vi "test - Clear CSM Queue.vi"(8 "error in (no error)":errorcluster, 11 "TestCase in":refnum<class "testcase-Basic-Function.lvclass">) -> (0 "error out":errorcluster, 3 "TestCase out":refnum<class "testcase-Basic-Function.lvclass">)   [LabVIEW 2017, in "testcase-Basic-Function.lvclass"]
uses:
  testcase-Basic-Function.lvclass
  src/user.lib/_NEVSTOP/Communicable State Machine(CSM)/_Support/CSMQ/_CSMOFGVOPER.ctl
  src/user.lib/_NEVSTOP/Communicable State Machine(CSM)/AdvanceAPI/CSM - Revert Arguments-Safe String.vi
  src/user.lib/_NEVSTOP/Communicable State Machine(CSM)/AdvanceAPI/CSM - Make String Arguments Safe.vi
  src/user.lib/_NEVSTOP/Communicable State Machine(CSM)/AdvanceAPI/CSM - Break Down Multiple States String.vi
  src/user.lib/_NEVSTOP/Communicable State Machine(CSM)/AdvanceAPI/CSM - Compact Multiple States.vi
  src/user.lib/_NEVSTOP/Communicable State Machine(CSM)/AdvanceAPI/CSM - Keywords.vi
  src/user.lib/_NEVSTOP/Communicable State Machine(CSM)/_Shared/Trim Single-line Text.vi
  <vilib>/addons/_JKI Toolkits/VI Tester/TestCase.llb/TestCase.lvclass
  src/user.lib/_NEVSTOP/Communicable State Machine(CSM)/Communicable State Machine.lvlib
  C:/Program Files (x86)/National Instruments/LabVIEW 2017/vi.lib/addons/_JKI Toolkits/VI Tester/TestCase.llb/TestCase.lvclass
panel:
  out "# pending insert":i32
  out "# pending remove":i32
  out "#Flushed":cluster{i32, i32}
  out "#elements in queue":i32
  out "error out 5":errorcluster
  out "error out 4":errorcluster
  out "error out 3":errorcluster
  out "error out 2":errorcluster
  out "error out 1":errorcluster
  out "State History":string
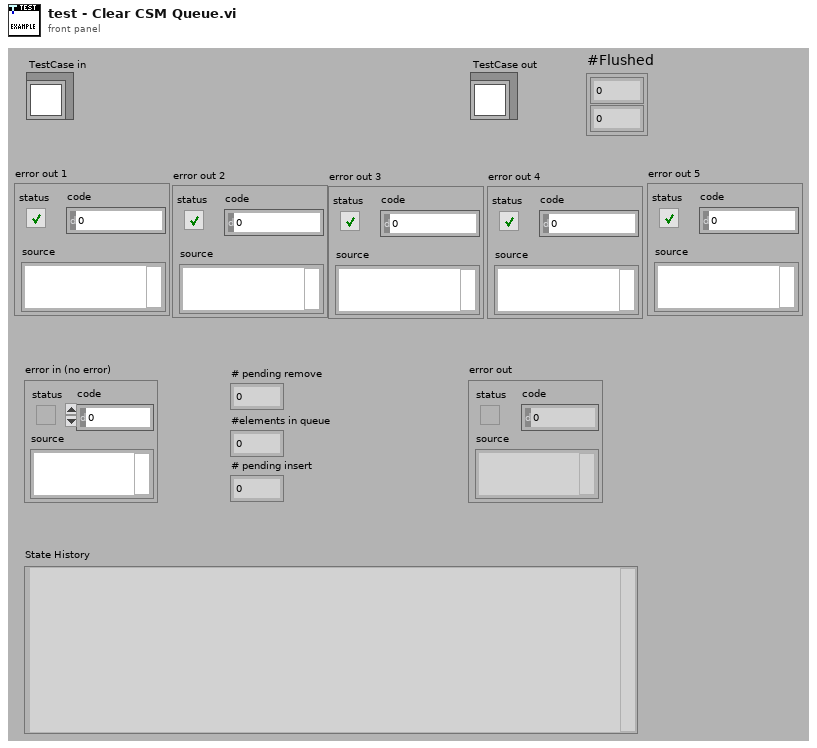
[diagram p1: front panel]
types:
  T1 = enum32{"Invalid", "Standard", "Closed", "Hidden", "Minimized", "Maximized"}
  T2 = enum32{"invalid app kind", "Development System", "Run Time System", "Student Edition", "Embedded LabVIEW", "Evaluation", "Custom"}
  T3 = typedef "Communicable State Machine.lvlib/_CSMOFGVOPER.ctl" = enum16{"Create If not Exist", "Get By Name", "List", "Check If Name Exists", "Release", "Module Status", "Create Status Event Handler", "Destroy Status Event Handler", "Clear Invalid Objs"}
  T4 = typedef "Communicable State Machine.lvlib/_CSM_Response Source Message.ctl" = cluster{"‘State":string, "’Arguments":string, "’Error":errorcluster}
  T5 = cluster{"Current VI Reference":refnum<vi>, "Close Panel on Exit?":bool}
  T6 = cluster{"Core":cluster{"Current VI Reference":refnum<vi>, "Close Panel on Exit?":bool}, "Your Boolean data":bool, "Your string data":string}
  T7 = typedef "Communicable State Machine.lvlib/_CSMObj.ctl" = cluster{"info":T8, "Refs":T10}
  T8 = typedef "Communicable State Machine.lvlib/_CSMObj-Info.ctl" = cluster{"Module Name":string, "Requested Name":string, "Group Name":string, "Mode":T9, "Allowed Messages":string[]}
  T9 = typedef "Communicable State Machine.lvlib/_CSM_MODE.ctl" = enum16{"Not Exist", "Stand Alone", "CSM", "Worker", "Worker Agent", "Chain Node", "Chain"}
  T10 = typedef "Communicable State Machine.lvlib/_CSMObj-Refs.ctl" = cluster{"WatchDogQ":refnum<queue>, "CSMDataDVR":refnum<data-value>, "Queue":T11, "GroupDataDVR":refnum<data-value>, "TagMap":refnum<data-value>, "ExitEvent":refnum<user-event>, "NewStateEvent":refnum<user-event>, "StatusEvent":refnum<user-event>, "InterruptEvent":refnum<user-event>}
  T11 = typedef "Communicable State Machine.lvlib/Priority Queue.ctl" = cluster{"HPriorityQ":refnum<queue>, "LowPriorityQ":refnum<queue>}
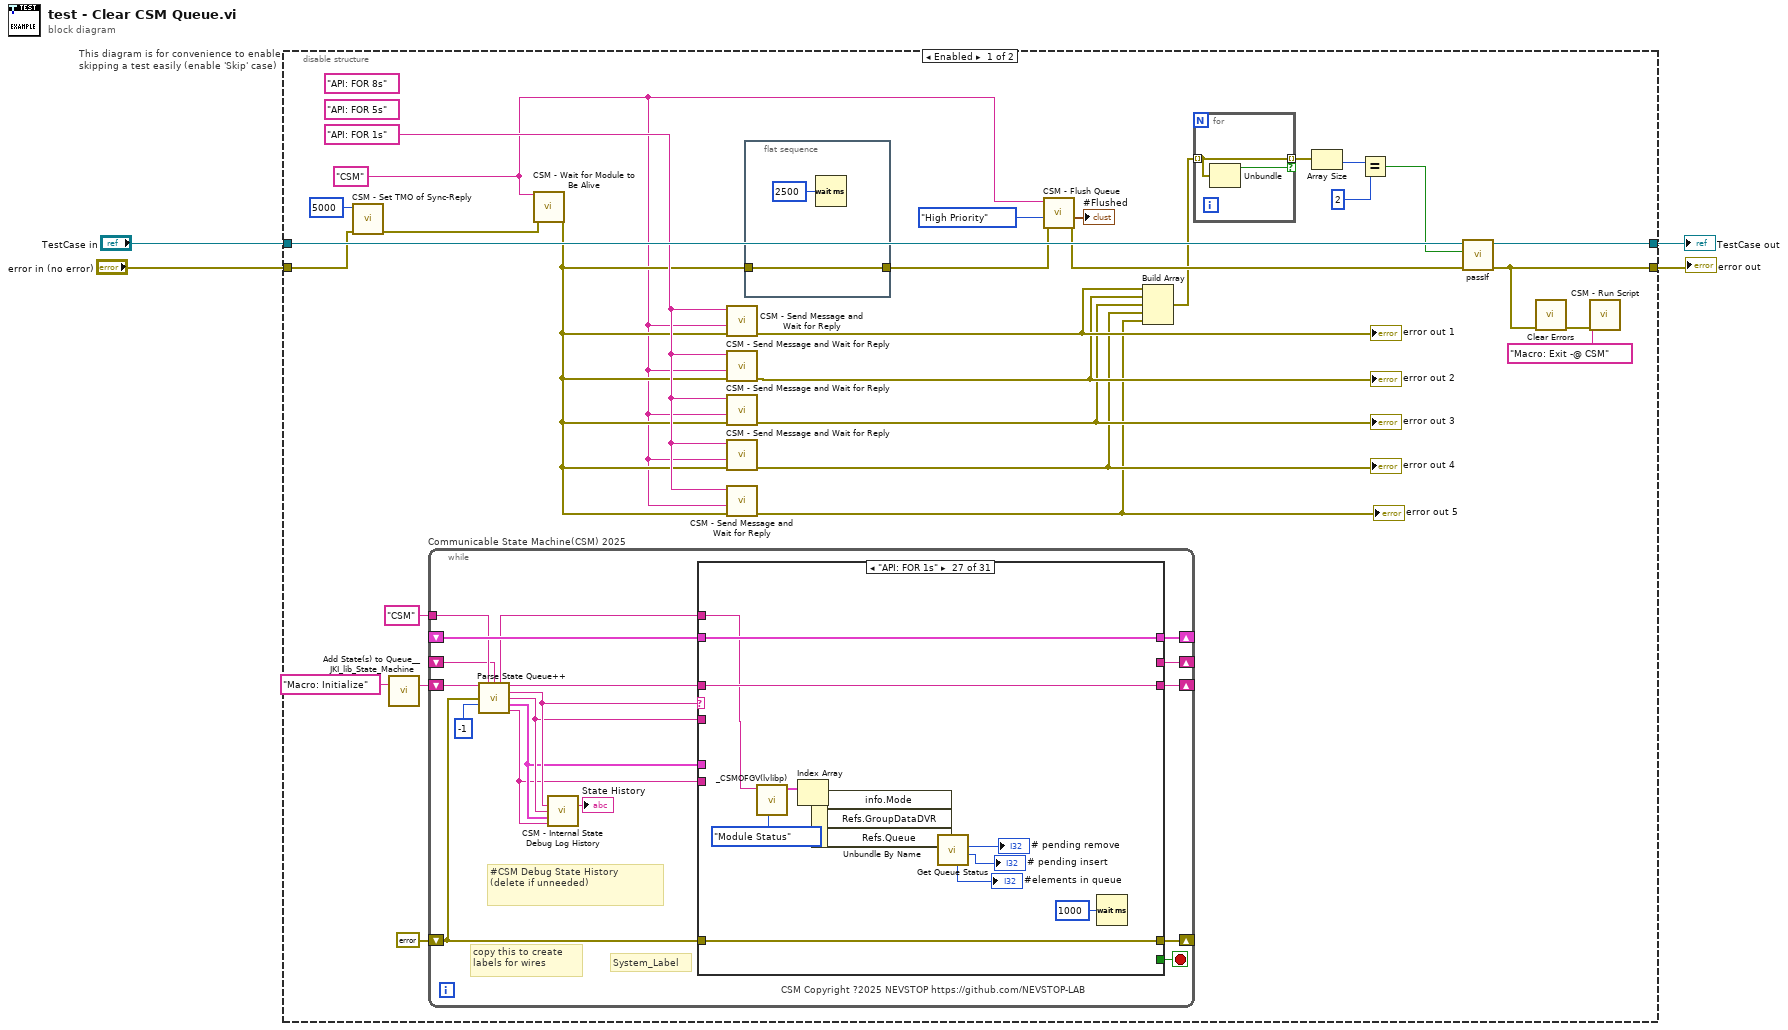
[diagram p0: block diagram]
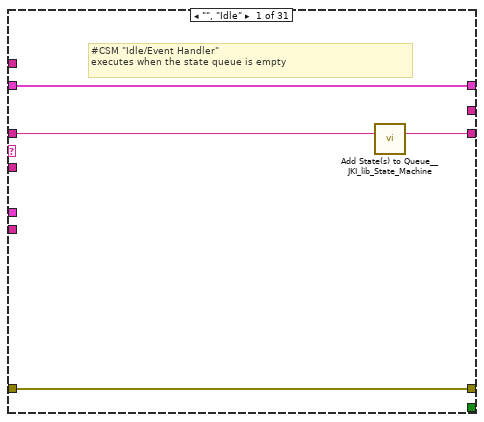
[diagram p2: hidden frame]
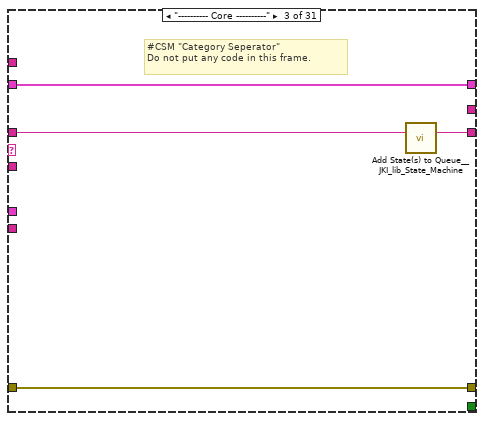
[diagram p4: hidden frame]
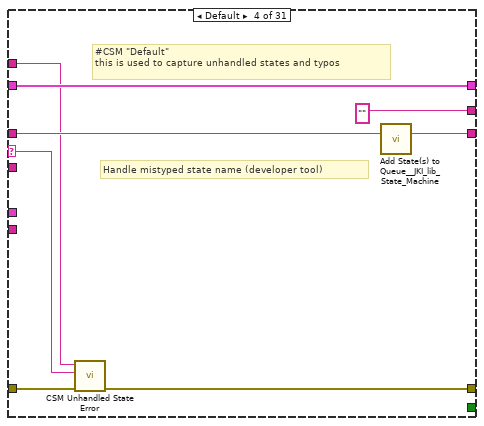
[diagram p5: hidden frame]
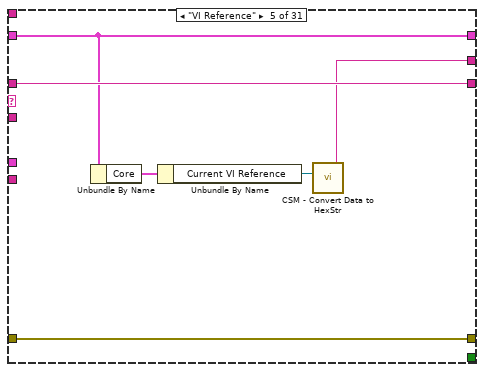
[diagram p6: hidden frame]
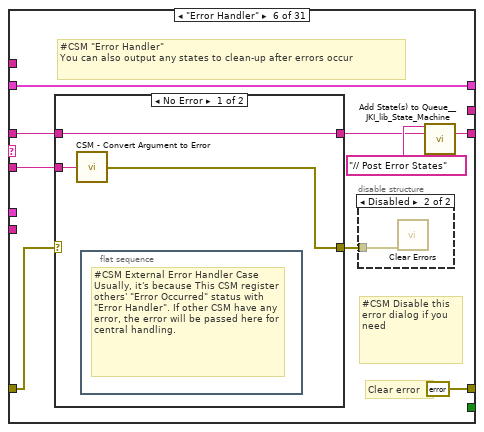
[diagram p7: hidden frame]
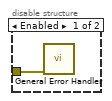
[diagram p8: hidden frame]
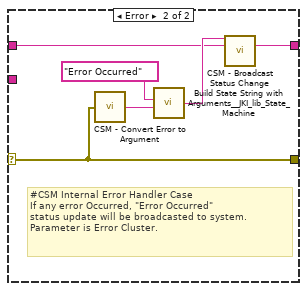
[diagram p9: hidden frame]
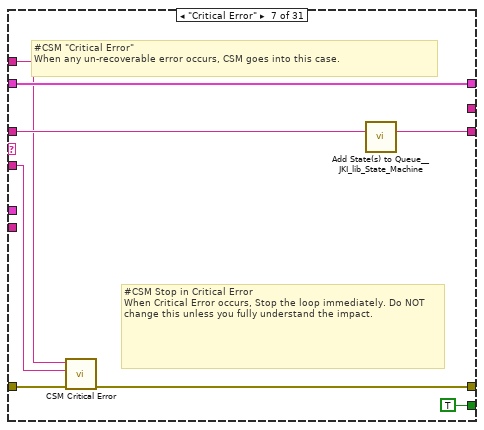
[diagram p10: hidden frame]
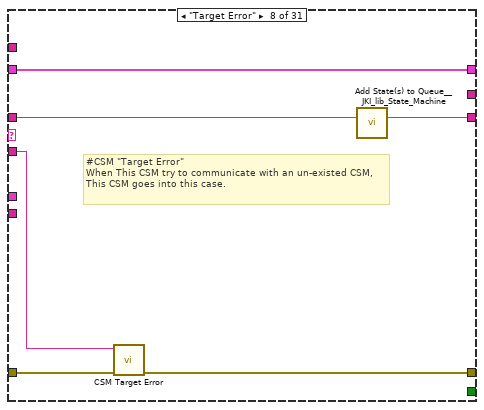
[diagram p11: hidden frame]
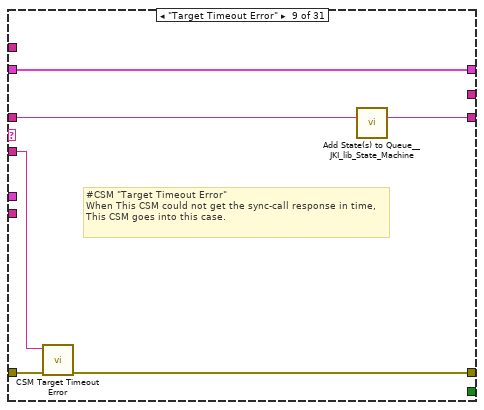
[diagram p12: hidden frame]
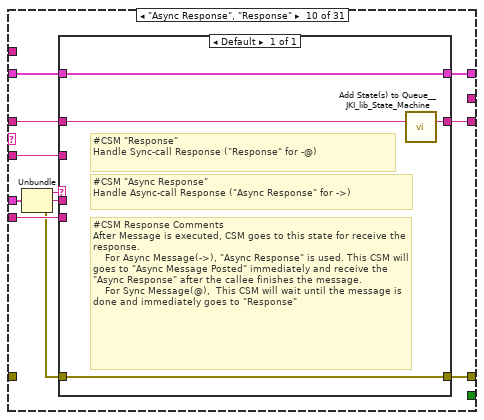
[diagram p13: hidden frame]
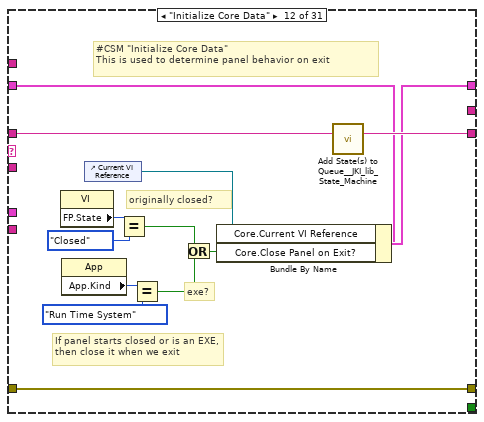
[diagram p15: hidden frame]
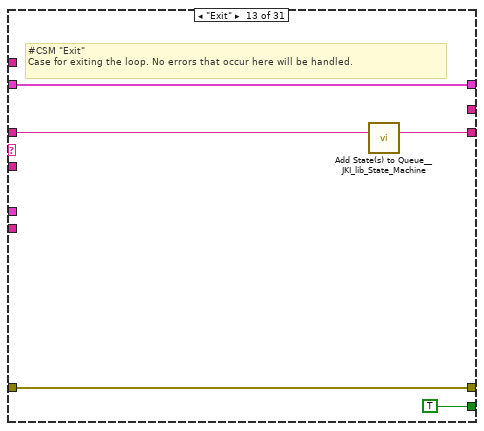
[diagram p16: hidden frame]
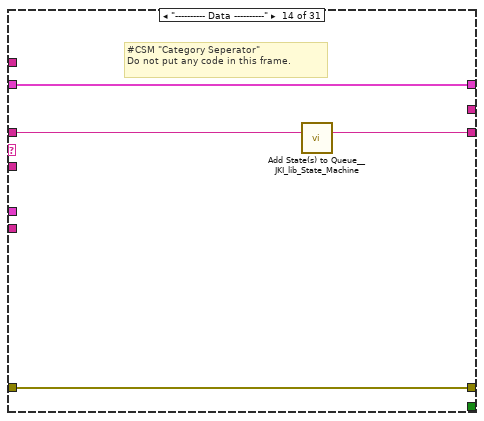
[diagram p17: hidden frame]
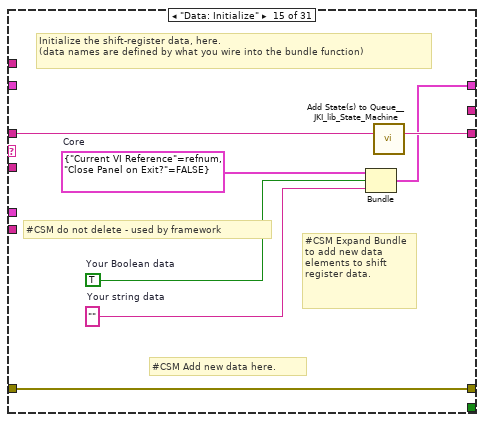
[diagram p18: hidden frame]
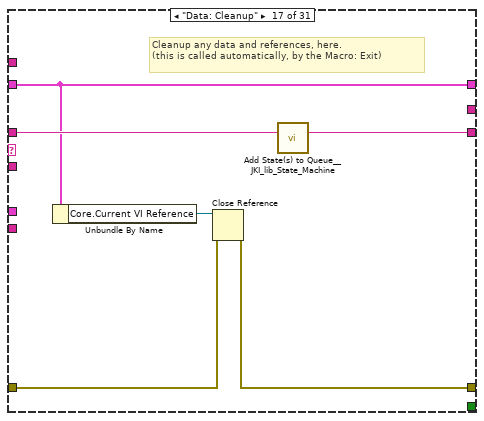
[diagram p20: hidden frame]
diagram:
  n1 = disable-structure "This diagram is for convenience to enable skipping a test easily (enable 'Skip' case)" shown="Enabled" {
    disable-tunnel: "TestCase in" -> [w25 w325]
    disable-tunnel: [w29 w323] -> w1
    disable-tunnel: [w28 w324] -> w3
    disable-tunnel: "error in (no error)" -> [w8 w322]
    frame Enabled {
      (unwired) "API: FOR 8s" ("State")
      (unwired) "API: FOR 5s" ("State")
      w24 = "API: FOR 1s" ("State")
      w20 = "CSM" ("Name (\"\" to Use UUID)")
      n2 = call "CSM - Set TMO of Sync-Reply.vi"("Error In"=w8, "TMO For Sync-Rep (ms) In"=5000 ("TMO for Sync-Rep(ms) In")) -> ("error out"=w7:errorcluster)  [unwired: 8 in, 1 out]
      n3 = call <vilib>:"Add State(s) to Queue__JKI_lib_State_Machine.vi"("State(s) in (\"\")"="Macro: Initialize" ("Init State(\"Macro: Initialize\")")) -> ("States Out"=w33:string)  [unwired: 14 in]
      n4 = while "Communicable State Machine(CSM) 2025" {
        shift-right: [w50] -> _
        shift-left: _ -> [w49]
        shift-right: [w53] -> _
        shift-left: errorcluster {"status"=FALSE, "code"=0, "source"=""} ("error out") -> [w48]
        shift-right: [w52] -> _
        shift-left: w33 -> [w54]
        tunnel: "CSM" ("Name (\"\" to Use UUID)") -> [w46]
        shift-right: [w47] -> _
        shift-left: _ -> [w40]
        stop <- w51 stop-if-true
        # "#CSM Debug State History\n(delete if unneeded)"
        # "copy this to create labels for wires"
        # "System_Label"
        # "CSM Copyright ?2025 NEVSTOP https://github.com/NEVSTOP-LAB"
        n5 = call "Parse State Queue++.vi"("State Queue"=w54, "Name (\"\" to Use UUID)"=w46, "Response Arguments"=w40, "Previous Error"=w48, "Dequeue (1 ms)"=-1 ("Timeout")) -> ("Name Used"=w41:string, "Remaining States"=w55:string, "Current State"=w45:string, "Arguments"=w44:string, "Additional Information"=w43:T4, "Source CSM"=w42:string)  [unwired: 5 in]
        n6 = call "CSM - Internal State Debug Log History.vi"("State"=w45, "Arguments (\"\")"=w44, ">> Response Source Message >>"=w43, "Source (\"\")"=w42) -> ("Debug Log"=→"State History":string)  [unwired: 11 in]
        n7 = case shown="\"API: FOR 1s\"" w45 {
          selector: w45 -> [_ _ _ w69 _ _ _ _ _ _ _ _ _ _ _ _ _ _ _ _ _ _ _ _ _ _ _ _ _ _ _]
          tunnel: w55 -> [w56 w61 w66 w73 w79 w85 w106 w112 w118 w126 w137 w151 w156 w160 w167 w169 w176 w180 w184 w190 w205 w274 w279 w286 w288 w292 w304 w308 w313 w317 w321]
          tunnel: w44 -> [_ _ _ _ _ w84 w102 w111 w116 w125 _ _ _ _ _ _ _ _ _ w185 w199 _ _ _ _ _ _ _ _ _ _]
          tunnel: w49 -> [w57 w60 w63 w71 w78 w88 w107 w113 w119 w128 w136 w144 w154 w157 _ w168 w171 w177 w182 w188 w201 w271 w276 w283 w287 w291 w303 w307 w310 w314 w318]
          tunnel: [w58 w62 w64 w67 w80 errorcluster {"status"=FALSE, "code"=0, "source"=""} ("error out") w103 w109 w115 w131 w138 w148 w153 w158 w164 w170 w172 w178 w181 w186 w202 w272 w277 w284 w289 w293 w305 w309 w311 w315 w319] -> w53
          tunnel: w48 -> [w58 w62 w64 w74 w80 w86 w108 w110 w117 _ w138 w148 w153 w158 w164 w170 w173 w178 w181 w187 w203 w272 w277 w284 w289 w293 w305 w309 w311 w315 w319]
          tunnel: [w59 w61 w65 w72 w79 w81 w105 w114 w120 w127 w137 w150 w155 w159 w166 w169 w175 w179 w183 w189 w204 w273 w278 w285 w288 w292 w304 w308 w312 w316 w320] -> w52
          tunnel: [_ _ _ _ _ _ TRUE _ _ _ _ _ TRUE _ _ _ _ _ _ _ _ _ _ _ _ _ _ _ _ _ _] -> w51
          tunnel: [w57 w60 w63 w71 w78 w88 w107 w113 w119 w129 w136 w149 w154 w157 w165 w168 w171 w177 w182 w188 w201 w271 w276 w283 w287 w291 w303 w307 w310 w314 w318] -> w50
          tunnel: w42 -> [_ _ _ _ _ _ _ _ _ w123 _ _ _ _ _ _ _ _ _ _ _ _ _ _ _ _ _ _ _ _ _]
          tunnel: w43 -> [_ _ _ _ _ _ _ _ _ w130 _ _ _ _ _ _ _ _ _ _ _ _ _ _ _ _ _ _ _ _ _]
          tunnel: [_ _ _ "" w75 _ _ _ _ _ _ _ _ _ _ _ _ _ _ _ _ _ _ _ _ _ _ _ _ _ _] -> w47
          tunnel: w41 -> [_ _ _ w68 _ _ w101 _ _ _ _ _ _ _ _ _ _ _ _ _ _ _ _ _ _ _ w300 _ _ _ _]
          frame "", "Idle" {
            # "#CSM \"Idle/Event Handler\"\nexecutes when the state queue is empty"
            n8 = call <vilib>:"Add State(s) to Queue__JKI_lib_State_Machine.vi"("State(s) in (\"\")"=w56) -> ("States Out"=w59:string)  [unwired: 14 in]
          }
          frame "CSM Documentation" {
            # "#CSM README FIRST\n\nCommunicable State Machine(CSM) is a LabVIEW application framework that builds upon JKI State Machine(JKISM). It follows the pattern of JKISM and extends the keywords to describe message communication between modules, including concepts such as Sync-Message, Async-Message, Subscription/Unsubscription of status - essential elements for creating reusable code modules. For more information, please visit the CSM wiki: https://nevstop-lab.github.io/CSM-Wiki/\n\nFor instructions on JKI State Machine, visit: http://jki.net/state-machine/\nFor information about CSM, visit: https://github.com/NEVSTOP-LAB"
            # "#CSM \"Documentation\"\nCase for holding CSM Documenation"
          }
          frame "---------- Core ----------" {
            # "#CSM \"Category Seperator\"\nDo not put any code in this frame."
            n9 = call <vilib>:"Add State(s) to Queue__JKI_lib_State_Machine.vi"("State(s) in (\"\")"=w66) -> ("States Out"=w65:string)  [unwired: 14 in]
          }
          frame Default {
            # "#CSM \"Default\"\nthis is used to capture unhandled states and typos"
            # "Handle mistyped state name (developer tool)"
            n10 = call "CSM Unhandled State Error.vi"("error in (no error)"=w74, "Undefined State"=w69, "CSM Name"=w68) -> ("error out"=w67:errorcluster)  [unwired: 8 in]
            n11 = call <vilib>:"Add State(s) to Queue__JKI_lib_State_Machine.vi"("State(s) in (\"\")"=w73) -> ("States Out"=w72:string)  [unwired: 14 in]
          }
          frame "VI Reference" {
            n12 = Unbundle By Name(w78) -> ("Core"=w77:T5)
            n13 = Unbundle By Name(w77) -> ("Current VI Reference"=w76:refnum<vi>)
            n14 = call "CSM - Convert Data to HexStr.vi"("Variant"=w76) -> ("HEX String (0-9,A-F)"=w75:string)  [unwired: 8 in]
          }
          frame "Error Handler" {
            # "#CSM Disable this error dialog if you need"
            # "#CSM \"Error Handler\"\nYou can also output any states to clean-up after errors occur"
            # "Clear error"
            n15 = case shown="No Error" w86 {
              selector: w86 -> [_ w95]
              tunnel: [w94 w97] -> w82
              tunnel: w85 -> [w94 w96]
              tunnel: w84 -> [w93 _]
              tunnel: [w92 w95] -> w87
              frame No Error {
                n16 = call "CSM - Convert Argument to Error.vi"("Argument"=w93) -> ("Error"=w92:errorcluster)  [unwired: 4 in]
                n17 = flat-sequence {
                  frame #0 {
                    # "#CSM External Error Handler Case\nUsually, it's because This CSM register others' \"Error Occurred\" status with \"Error Handler\". If other CSM have any error, the error will be passed here for central handling."
                  }
                }
              }
              frame Error {
                # "#CSM Internal Error Handler Case \nIf any error Occurred, \"Error Occurred\" \nstatus update will be broadcasted to system.\nParameter is Error Cluster."
                n18 = call "CSM - Convert Error to Argument.vi"("Error"=w95) -> ("Argument"=w99:string)  [unwired: 4 in]
                n19 = call <vilib>:"Build State String with Arguments__JKI_lib_State_Machine.vi"("Arguments (\"\")"=w99, "State"="Error Occurred" ("Status with Arguments")) -> ("State with Arguments"=w98:string)  [unwired: 4 in]
                n20 = call "CSM - Broadcast Status Change.vi"("Status With Arguments"=w98, "State Queue"=w96) -> ("Remaining States"=w97:string)  [unwired: 13 in]
              }
            }
            n21 = disable-structure shown="Disabled" {
              disable-tunnel: w87 -> [w90 w91]
              frame Enabled {
                n22 = call <vilib>:"General Error Handler.vi"("error in (no error)"=w90) -> ()  [unwired: 10 in, 5 out]
              }
              frame Disabled {
                n23 = call <vilib>:"Clear Errors.vi"("error in (no error)"=w91) -> ()  [unwired: 5 in, 2 out]
              }
            }
            n24 = call <vilib>:"Add State(s) to Queue__JKI_lib_State_Machine.vi"("State(s) in Front (\"\")"="// Post Error States", "State(s) in (\"\")"=w82) -> ("States Out"=w81:string)  [unwired: 13 in]
          }
          frame "Critical Error" {
            # "#CSM Stop in Critical Error\nWhen Critical Error occurs, Stop the loop immediately. Do NOT change this unless you fully understand the impact."
            # "#CSM \"Critical Error\"\nWhen any un-recoverable error occurs, CSM goes into this case."
            n25 = call "CSM Critical Error.vi"("error in (no error)"=w108, "Arugments (As Reason)"=w102, "CSM Name"=w101) -> ("error out"=w103:errorcluster)  [unwired: 8 in]
            n26 = call <vilib>:"Add State(s) to Queue__JKI_lib_State_Machine.vi"("State(s) in (\"\")"=w106) -> ("States Out"=w105:string)  [unwired: 14 in]
          }
          frame "Target Error" {
            # "#CSM \"Target Error\"\nWhen This CSM try to communicate with an un-existed CSM, This CSM goes into this case."
            n27 = call "CSM Target Error.vi"("error in (no error)"=w110, "Arguments (As CSM Name)"=w111) -> ("error out"=w109:errorcluster)  [unwired: 9 in]
            n28 = call <vilib>:"Add State(s) to Queue__JKI_lib_State_Machine.vi"("State(s) in (\"\")"=w112) -> ("States Out"=w114:string)  [unwired: 14 in]
          }
          frame "Target Timeout Error" {
            # "#CSM \"Target Timeout Error\"\nWhen This CSM could not get the sync-call response in time, This CSM goes into this case."
            n29 = call "CSM Target Timeout Error.vi"("error in (no error)"=w117, "Arguments (As CSM Name)"=w116) -> ("error out"=w115:errorcluster)  [unwired: 9 in]
            n30 = call <vilib>:"Add State(s) to Queue__JKI_lib_State_Machine.vi"("State(s) in (\"\")"=w118) -> ("States Out"=w120:string)  [unwired: 14 in]
          }
          frame "Async Response", "Response" {
            n31 = Unbundle(w130) -> ("‘State"=w124:string, "’Arguments"=w122:string, "’Error"=w121:errorcluster)
            n32 = case shown="Default" w124 {
              tunnel: [w135] -> w131
              tunnel: w121 -> [w135]
              tunnel: [w134] -> w129
              tunnel: w128 -> [w134]
              tunnel: [w132] -> w127
              tunnel: w126 -> [w133]
              tunnel: w125 -> [_]
              tunnel: w123 -> [_]
              tunnel: w122 -> [_]
              frame Default {
                # "#CSM Response Comments\nAfter Message is executed, CSM goes to this state for receive the response.\n    For Async Message(->), \"Async Response\" is used. This CSM will goes to \"Async Message Posted\" immediately and receive the \"Async Response\" after the callee finishes the message.\n    For Sync Message(@),  This CSM will wait until the message is done and immediately goes to \"Response\""
                # "#CSM \"Async Response\"\nHandle Async-call Response (\"Async Response\" for ->)"
                # "#CSM \"Response\"\nHandle Sync-call Response (\"Response\" for -@)"
                n33 = call <vilib>:"Add State(s) to Queue__JKI_lib_State_Machine.vi"("State(s) in (\"\")"=w133) -> ("States Out"=w132:string)  [unwired: 14 in]
              }
            }
          }
          frame "Async Message Posted" {
            # "#CSM \"Async Message Posted\"\nAfter Async Message is posted (-> or ->| ), CSM goes to this state for post-action.\nYou can use Argument - State to tell which Async Message is called."
          }
          frame "Initialize Core Data" {
            # "#CSM \"Initialize Core Data\"\nThis is used to determine panel behavior on exit"
            # "originally closed?"
            # "exe?"
            # "If panel starts closed or is an EXE, then close it when we exit"
            n34 = property class="VI"() -> ("FP.State"=w141:T1)  [unwired: 2 in, 2 out]
            n35 = property class="App"() -> ("App.Kind"=w147:T2)  [unwired: 2 in, 2 out]
            n36 = control-ref of="Current VI Reference"() -> (w142:refnum<vi>)
            n37 = Equal?(x=w141, y=T1."Closed" ("Front Panel Window:State")) -> (x = y?=w139:bool)
            n38 = Equal?(x=w147, y=T2."Run Time System" ("Application:Kind")) -> (x = y?=w145:bool)
            n39 = Or(x=w139, y=w145) -> (x .or. y?=w143:bool)
            n40 = Bundle By Name(cluster=w144, "Core.Current VI Reference"=w142, "Core.Close Panel on Exit?"=w143) -> (w149:T6)
            n41 = call <vilib>:"Add State(s) to Queue__JKI_lib_State_Machine.vi"("State(s) in (\"\")"=w151) -> ("States Out"=w150:string)  [unwired: 14 in]
          }
          frame "Exit" {
            # "#CSM \"Exit\"\nCase for exiting the loop. No errors that occur here will be handled."
            n42 = call <vilib>:"Add State(s) to Queue__JKI_lib_State_Machine.vi"("State(s) in (\"\")"=w156) -> ("States Out"=w155:string)  [unwired: 14 in]
          }
          frame "---------- Data ----------" {
            # "#CSM \"Category Seperator\"\nDo not put any code in this frame."
            n43 = call <vilib>:"Add State(s) to Queue__JKI_lib_State_Machine.vi"("State(s) in (\"\")"=w160) -> ("States Out"=w159:string)  [unwired: 14 in]
          }
          frame "Data: Initialize" {
            w161 = T5 {"Current VI Reference"=refnum, "Close Panel on Exit?"=FALSE}  # Core
            w163 = TRUE  # Your Boolean data
            w162 = ""  # Your string data
            # "#CSM do not delete - used by framework"
            # "#CSM Expand Bundle to add new data elements to shift register data."
            # "#CSM Add new data here."
            # "Initialize the shift-register data, here.\n(data names are defined by what you wire into the bundle function)"
            n44 = Bundle("Core"=w161, "Your Boolean data"=w163, "Your string data"=w162) -> (w165:T6)  [unwired: 1 in]
            n45 = call <vilib>:"Add State(s) to Queue__JKI_lib_State_Machine.vi"("State(s) in (\"\")"=w167) -> ("States Out"=w166:string)  [unwired: 14 in]
          }
          frame "Data: Update Indicators" {
          }
          frame "Data: Cleanup" {
            # "Cleanup any data and references, here.\n(this is called automatically, by the Macro: Exit)"
            n46 = Unbundle By Name(w171) -> ("Core.Current VI Reference"=w174:refnum<vi>)
            n47 = Close Reference(reference=w174, error in (no error)=w173) -> (error out=w172:errorcluster)
            n48 = call <vilib>:"Add State(s) to Queue__JKI_lib_State_Machine.vi"("State(s) in (\"\")"=w176) -> ("States Out"=w175:string)  [unwired: 14 in]
          }
          frame "---------- UI ----------" {
            # "#CSM \"Category Seperator\"\nDo not put any code in this frame."
            n49 = call <vilib>:"Add State(s) to Queue__JKI_lib_State_Machine.vi"("State(s) in (\"\")"=w180) -> ("States Out"=w179:string)  [unwired: 14 in]
          }
          frame "UI: Initialize" {
            # "#CSM \"UI: Initialize\"\nInitialize the User Interface, here.\n(this is called automatically, by the Macro: Init)"
            n50 = call <vilib>:"Add State(s) to Queue__JKI_lib_State_Machine.vi"("State(s) in (\"\")"=w184) -> ("States Out"=w183:string)  [unwired: 14 in]
          }
          frame "UI: Cursor Set" {
            # "#CSM \"UI: Cursor Set\"\nSet and Unset Cursor Busy.\n(Usage: \"UI: Cursor Set >> Busy|Idle\")"
            # "Argument"
            n51 = disable-structure shown="TARGET_TYPE!=Windows" {
              disable-tunnel: w187 -> [w193 w198]
              disable-tunnel: [w192 w198] -> w186
              disable-tunnel: w185 -> [w191 _]
              frame condition #0 (active) {
                n52 = case shown="\"Idle\", Default" w191 {
                  tunnel: w193 -> [w195 w197]
                  tunnel: [w194 w196] -> w192
                  frame "Idle", Default {
                    n53 = call <vilib>:"Unset Busy.vi"("error in (no error)"=w195) -> ("error out"=w194:errorcluster)  [unwired: 10 in]
                  }
                  frame "Busy" {
                    n54 = call <vilib>:"Set Busy.vi"("error in (no error)"=w197) -> ("error out"=w196:errorcluster)  [unwired: 9 in, 1 out]
                  }
                }
              }
              frame condition #1 {
              }
            }
            n55 = call <vilib>:"Add State(s) to Queue__JKI_lib_State_Machine.vi"("State(s) in (\"\")"=w190) -> ("States Out"=w189:string)  [unwired: 14 in]
          }
          frame "UI: Front Panel State" {
            # "#CSM \"UI: Front Panel State\"\nSet Front Panel Open or Closed\n(Usage: \"UI: Front Panel State >> Open|Close\")"
            # "Argument"
            n56 = Unbundle By Name(w201) -> ("Core.Current VI Reference"=w200:refnum<vi>)
            n57 = call <vilib>:"Add State(s) to Queue__JKI_lib_State_Machine.vi"("State(s) in (\"\")"=w205) -> ("States Out"=w204:string)  [unwired: 14 in]
            n58 = case shown="\"Close\", \"Closed\"" w199 {
              tunnel: w203 -> [w211 w226 w237 w250 w263]
              tunnel: [w213 w227 w239 w252 w265] -> w202
              tunnel: w200 -> [w212 w224 w238 w251 w264]
              frame "Open", "Standard", Default {
                w206 = T1."Standard" ("State")
                n59 = property class="VI"(reference=w212, error in=w211) -> (reference out=w209:refnum<vi>, error out=w210:errorcluster, "FP.State"=w208:T1)
                n60 = Not Equal?(x=w208, y=w206) -> (x != y?=w207:bool)
                n61 = case shown="True" w207 {
                  tunnel: [w217 w219] -> w213
                  tunnel: w210 -> [w216 w219]
                  tunnel: w209 -> [w215 _]
                  tunnel: w206 -> [w214 _]
                  frame True {
                    n62 = invoke class="VI" method="FP.Open"(reference=w215, error in=w216, "Activate"=TRUE, "State"=w214) -> (error out=w217:errorcluster)  [unwired: 1 in, 4 out]
                  }
                  frame False {
                  }
                }
              }
              frame "Close", "Closed" {
                n63 = property class="VI"(reference=w224, error in=w226) -> (reference out=w223:refnum<vi>, error out=w225:errorcluster, "FP.State"=w221:T1)
                n64 = Not Equal?(x=w221, y=T1."Closed" ("Front Panel Window:State")) -> (x != y?=w220:bool)
                n65 = case shown="False" w220 {
                  tunnel: [w228 w231] -> w227
                  tunnel: w225 -> [w228 w230]
                  tunnel: w223 -> [_ w229]
                  frame False {
                  }
                  frame True {
                    n66 = invoke class="VI" method="FP.Close"(reference=w229, error in=w230) -> (error out=w231:errorcluster)  [unwired: 1 in, 2 out]
                  }
                }
              }
              frame "Hidden", "Hide" {
                w232 = T1."Hidden" ("State")
                n67 = property class="VI"(reference=w238, error in=w237) -> (reference out=w235:refnum<vi>, error out=w236:errorcluster, "FP.State"=w234:T1)
                n68 = Not Equal?(x=w234, y=w232) -> (x != y?=w233:bool)
                n69 = case shown="True" w233 {
                  tunnel: [w243 w244] -> w239
                  tunnel: w236 -> [w242 w244]
                  tunnel: w235 -> [w241 _]
                  tunnel: w232 -> [w240 _]
                  frame True {
                    n70 = invoke class="VI" method="FP.Open"(reference=w241, error in=w242, "State"=w240) -> (error out=w243:errorcluster)  [unwired: 2 in, 4 out]
                  }
                  frame False {
                  }
                }
              }
              frame "Minimize", "Minimized" {
                w245 = T1."Minimized" ("State")
                n71 = property class="VI"(reference=w251, error in=w250) -> (reference out=w248:refnum<vi>, error out=w249:errorcluster, "FP.State"=w247:T1)
                n72 = Not Equal?(x=w247, y=w245) -> (x != y?=w246:bool)
                n73 = case shown="True" w246 {
                  tunnel: [w256 w257] -> w252
                  tunnel: w249 -> [w255 w257]
                  tunnel: w248 -> [w254 _]
                  tunnel: w245 -> [w253 _]
                  frame True {
                    n74 = invoke class="VI" method="FP.Open"(reference=w254, error in=w255, "State"=w253) -> (error out=w256:errorcluster)  [unwired: 2 in, 4 out]
                  }
                  frame False {
                  }
                }
              }
              frame "Maximize", "Maximized" {
                w258 = T1."Maximized" ("State")
                n75 = property class="VI"(reference=w264, error in=w263) -> (reference out=w261:refnum<vi>, error out=w262:errorcluster, "FP.State"=w260:T1)
                n76 = Not Equal?(x=w260, y=w258) -> (x != y?=w259:bool)
                n77 = case shown="True" w259 {
                  tunnel: [w269 w270] -> w265
                  tunnel: w262 -> [w268 w270]
                  tunnel: w261 -> [w267 _]
                  tunnel: w258 -> [w266 _]
                  frame True {
                    n78 = invoke class="VI" method="FP.Open"(reference=w267, error in=w268, "State"=w266) -> (error out=w269:errorcluster)  [unwired: 2 in, 4 out]
                  }
                  frame False {
                  }
                }
              }
            }
          }
          frame "---------- Macro ----------" {
            # "#CSM \"Category Seperator\"\nDo not put any code in this frame."
            n79 = call <vilib>:"Add State(s) to Queue__JKI_lib_State_Machine.vi"("State(s) in (\"\")"=w274) -> ("States Out"=w273:string)  [unwired: 14 in]
          }
          frame "Macro: Initialize" {
            # "#CSM \"Macro: Initialize\"\nInitialization Macro (This is called once, when the VI starts)"
            n80 = call <vilib>:"Add State(s) to Queue__JKI_lib_State_Machine.vi"("State(s) in Front (\"\")"="Data: Initialize\nInitialize Core Data\nData: Update Indicators", "State(s) in (\"\")"=w279) -> ("States Out"=w278:string)  [unwired: 13 in]
          }
          frame "Macro: Exit" {
            # "#CSM \"Macro: Exit\"\nExit Macro (This is called once, when the VI exits)"
            n81 = call <vilib>:"Add State(s) to Queue__JKI_lib_State_Machine.vi"("State(s) in Front (\"\")"="//Exit Sub-Modules ", "State(s) at Back (\"\")"="Data: Cleanup\nExit") -> ("States Out"=w281:string)  [unwired: 13 in]
            n82 = call <vilib>:"Add State(s) to Queue__JKI_lib_State_Machine.vi"("State(s) in Front (\"\")"=w281, "State(s) in (\"\")"=w286) -> ("States Out"=w285:string)  [unwired: 13 in]
          }
          frame "---------- API ----------" {
            # "#CSM \"Category Seperator\"\nDo not put any code in this frame."
          }
          frame "API: FOR 5s" {
            n83 = Wait (ms)(milliseconds to wait=u32 5000) -> ()  [unwired: 1 out]
          }
          frame "API: FOR 1s" {
            n84 = call "_CSMOFGV(lvlibp).vi"("Operation"=_CSMOFGVOPER."Module Status", "Name (\"\" to Use UUID) In"=w300) -> ("Array"=w298:T7[])  [unwired: 7 in, 2 out]
            n85 = Index Array(array=w298) -> (element=w299:T7)  [unwired: 1 in]
            n86 = Unbundle By Name(w299) -> ("Refs.Queue"=w297:T11)  [unwired: 2 out]
            n87 = call "Get Queue Status.vi"("Priority Queue In"=w297) -> ("# Pending Insert"=→"# pending insert":i32, "# Pending Remove"=→"# pending remove":i32, "# Elements In Queue"=→"#elements in queue":i32)  [unwired: 6 in, 2 out]
            n88 = Wait (ms)(milliseconds to wait=u32 1000) -> ()  [unwired: 1 out]
          }
          frame "API: FOR 8s" {
            n89 = Wait (ms)(milliseconds to wait=u32 8000) -> ()  [unwired: 1 out]
          }
          frame "---------- Action ----------" {
            # "#CSM \"Category Seperator\"\nDo not put any code in this frame."
            n90 = call <vilib>:"Add State(s) to Queue__JKI_lib_State_Machine.vi"("State(s) in (\"\")"=w313) -> ("States Out"=w312:string)  [unwired: 14 in]
          }
          frame "Action: action1" {
            # "#CSM \"Internal State\"\nThis category is used for holding internal states"
            n91 = call <vilib>:"Add State(s) to Queue__JKI_lib_State_Machine.vi"("State(s) in (\"\")"=w317) -> ("States Out"=w316:string)  [unwired: 14 in]
          }
          frame "Action: action2" {
            # "#CSM \"Internal State\"\nThis category is used for holding internal states"
            n92 = call <vilib>:"Add State(s) to Queue__JKI_lib_State_Machine.vi"("State(s) in (\"\")"=w321) -> ("States Out"=w320:string)  [unwired: 14 in]
          }
        }
      }
      n93 = call "CSM - Wait for Module to Be Alive.vi"("CSM Name"=w20, "error in (no error)"=w7) -> ("error out"=w22:errorcluster)  [unwired: 11 in, 2 out]
      n94 = call "CSM - Send Message and Wait for Reply.vi"("Error In (No Error)"=w22, "Target Module"=w20, "State"=w24) -> ("error out"=w18:errorcluster)  [unwired: 6 in, 2 out]
      "error out 1" <- w18
      n95 = call "CSM - Send Message and Wait for Reply.vi"("Error In (No Error)"=w22, "Target Module"=w20, "State"=w24) -> ("error out"=w17:errorcluster)  [unwired: 6 in, 2 out]
      "error out 2" <- w17
      n96 = call "CSM - Send Message and Wait for Reply.vi"("Error In (No Error)"=w22, "Target Module"=w20, "State"=w24) -> ("error out"=w16:errorcluster)  [unwired: 6 in, 2 out]
      "error out 3" <- w16
      n97 = call "CSM - Send Message and Wait for Reply.vi"("Error In (No Error)"=w22, "Target Module"=w20, "State"=w24) -> ("error out"=w15:errorcluster)  [unwired: 6 in, 2 out]
      "error out 4" <- w15
      n98 = call "CSM - Send Message and Wait for Reply.vi"("Error In (No Error)"=w22, "Target Module"=w20, "State"=w24) -> ("error out"=w14:errorcluster)  [unwired: 6 in, 2 out]
      "error out 5" <- w14
      n99 = flat-sequence {
        tunnel: [w36] -> w23
        tunnel: w22 -> [w36]
        frame #0 {
          n100 = Wait (ms)(milliseconds to wait=u32 2500) -> ()  [unwired: 1 out]
        }
      }
      n101 = call "CSM - Flush Queue.vi"("Error In"=w23, "Option (Low Priority As Default)"=enum16{"All", "High Priority", "Low Priority"}."High Priority" ("Option(Low Priority as Default)"), "CSM Name"=w20) -> ("error out"=w21:errorcluster, "#Flushed"=→"#Flushed":cluster{i32, i32})  [unwired: 6 in, 1 out]
      n102 = Build Array(w18, w17, w16, w15, w14) -> (w13:errorcluster[])
      n103 = for {
        tunnel: w13 -> [w35] mode=indexing
        tunnel: [w35] -> w12 mode=indexing if=w34
        n104 = Unbundle(w35) -> ("status"=w34:bool)  [unwired: 2 out]
      }
      n105 = Array Size(array=w12) -> (size(s)=w11:i32)
      n106 = Equal?(x=w11, y=2) -> (x = y?=w9:bool)
      n107 = call-dynamic "passIf.vi"("error in (no error)"=w21, "pass"=w9, "TestCase in"=w25) -> ("error out"=w28:errorcluster, "TestCase out"=w29:refnum<class "testcase-Basic-Function.lvclass">)  [unwired: 7 in]
      n108 = call <vilib>:"Clear Errors.vi"("error in (no error)"=w28) -> ("error out"=w27:errorcluster)  [unwired: 5 in, 1 out]
      n109 = call "CSM - Run Script.vi"("CSM Scripts"="Macro: Exit -@ CSM", "error in (no error)"=w27) -> ()  [unwired: 11 in, 3 out]
    }
    frame Disabled {
      # "skip test result while test is under development"
      n110 = call <vilib>:"skip.vi"("error in (no error)"=w322, "TestCase in"=w325) -> ("error out"=w324:errorcluster, "TestCase out"=w323:refnum<class "testcase-Basic-Function.lvclass">)  [unwired: 8 in]
    }
  }
  "error out" <- w3
  "TestCase out" <- w1
